vi "TCPserver.vi"(11 "Ref In":T1) -> ()   [LabVIEW 2016]
doc: "Demonstrates how to open a connection to an TCP server, read the data being sent, and display the data on a chart. This VI is designed to stop if the TCP connection is terminated."
panel:
  out "error out":errorcluster
  out "Current Pos":dbl[](array[numeric])
  in  "Position":dbl[](array[numeric])
  in  "Ring":u16(ring) items=["Move2Pos", "Move2Work", "ChangeManipulator", "Move2Home", "Calibration", "CurrentPos", "Interrupt"]
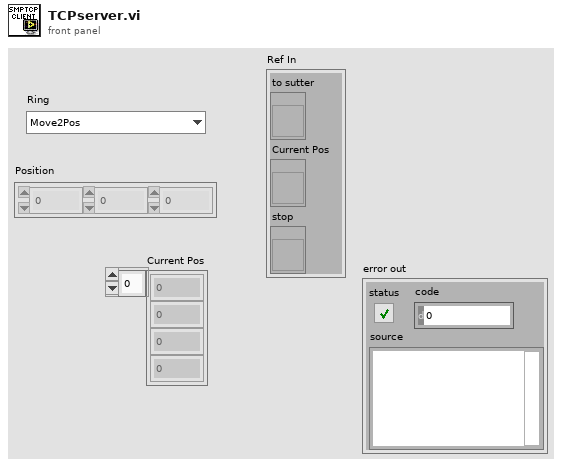
[diagram p1: front panel]
types:
  T1 = cluster{"to sutter":refnum<vi>, "Current Pos":refnum<vi>, "stop":refnum<vi>}
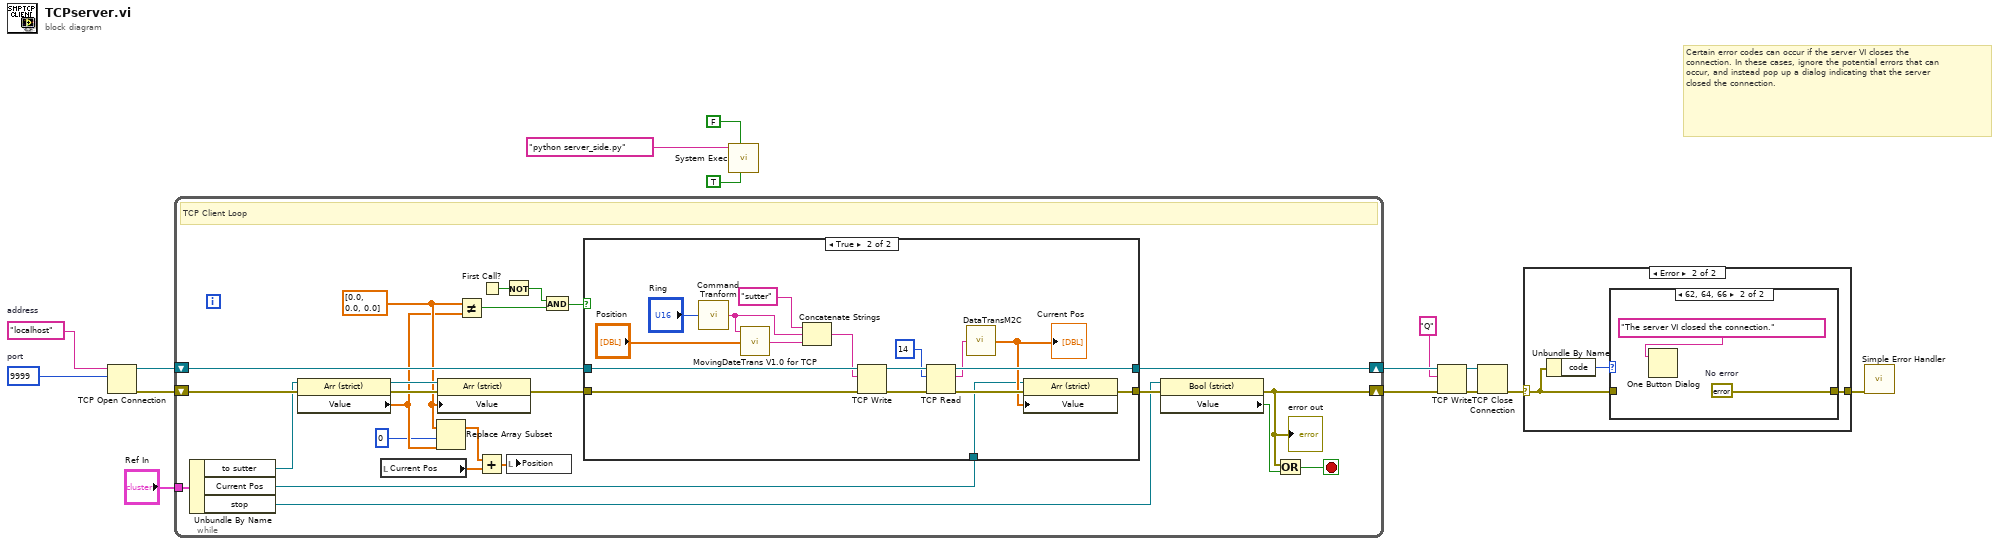
[diagram p0: block diagram]
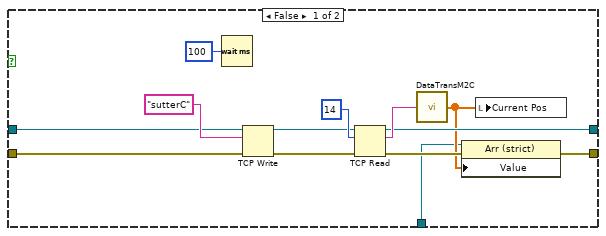
[diagram p4: hidden frame]
diagram:
  w7 = u16 9999  # port
  w8 = "localhost"  # address
  # "Certain error codes can occur if the server VI closes the connection. In these cases, ignore the potential errors that can occur, and instead pop up a dialog indicating that the server closed the connection."
  n1 = TCP Open Connection(address=w8, remote port or service name=w7) -> (connection ID=w5:refnum<k5>, error out=w4:errorcluster)  [unwired: 3 in]
  n2 = while {
    shift-right: [w34] -> w12
    shift-left: w4 -> [w39]
    shift-right: [w36] -> w14
    shift-left: w5 -> [w37]
    tunnel: "Ref In" -> [w27]
    stop <- w38 stop-if-true
    w19 = dbl[] [0.0, 0.0, 0.0] ("x")
    # "TCP Client Loop"
    n3 = Unbundle By Name(w27) -> ("to sutter"=w32:refnum<vi>, "Current Pos"=w20:refnum<vi>, "stop"=w21:refnum<vi>)
    n4 = property class="Arr (strict)"(reference=w32, error in=w39) -> (reference out=w30:refnum<vi>, error out=w29:errorcluster, "Value"=w18:sgl[])
    n5 = local read "Current Pos"() -> (w31:dbl[])
    n6 = Replace Array Subset(array=w19, new element=w18, index=0) -> (w17:dbl[])
    n7 = property class="Arr (strict)"(reference=w30, error in=w29, "Value"=w19) -> (error out=w28:errorcluster)  [unwired: 1 out]
    n8 = Not Equal?(x=w19, y=w18) -> (x != y?=w23:bool)
    n9 = Add(x=w17, y=w31) -> (x+y=w26:dbl[])
    n10 = First Call?() -> (First Call?: T/F=w25:bool)
    n11 = Not(x=w25) -> (.not. x?=w24:bool)
    n12 = local write "Position"(w26) -> ()
    n13 = And(x=w24, y=w23) -> (x .and. y?=w22:bool)
    n14 = case shown="True" w22 {
      tunnel: w37 -> [w46 w69]
      tunnel: [w44 w68] -> w36
      tunnel: [w42 w55] -> w35
      tunnel: w28 -> [w45 w57]
      tunnel: w20 -> [w40 w53]
      frame False {
        n15 = Wait (ms)(milliseconds to wait=u32 100) -> ()  [unwired: 1 out]
        n16 = TCP Write(connection ID=w46, data in="sutterC", error in (no error)=w45) -> (connection ID out=w49:refnum<k5>, error out=w48:errorcluster)  [unwired: 1 in, 1 out]
        n17 = TCP Read(connection ID=w49, bytes to read=14, error in (no error)=w48) -> (connection ID out=w44:refnum<k5>, data out=w51:string, error out=w43:errorcluster)  [unwired: 2 in]
        n18 = call "DataTransM2C.vi"("MotorData"=w51) -> ("Computer Data"=w41:dbl[])
        n19 = property class="Arr (strict)"(reference=w40, error in=w43, "Value"=w41) -> (error out=w42:errorcluster)  [unwired: 1 out]
        n20 = local write "Current Pos"(w41) -> ()
      }
      frame True {
        n21 = call "Command Tranform.vi"("Command"="Ring") -> ("command str"=w64:string)
        n22 = call "MovingDateTrans V1.0 for TCP.vi"("INPUT"="Position", "String"=w64) -> ("MOVEING COMMAND"=w66:string)  [unwired: 1 in]
        n23 = Concatenate Strings("sutter" ("string"), w64, w66) -> (w59:string)
        n24 = TCP Write(connection ID=w69, data in=w59, error in (no error)=w57) -> (connection ID out=w62:refnum<k5>, error out=w63:errorcluster)  [unwired: 1 in, 1 out]
        n25 = TCP Read(connection ID=w62, bytes to read=14, error in (no error)=w63) -> (connection ID out=w68:refnum<k5>, data out=w60:string, error out=w56:errorcluster)  [unwired: 2 in]
        n26 = call "DataTransM2C.vi"("MotorData"=w60) -> ("Computer Data"=w54:dbl[])
        "Current Pos" <- w54
        n27 = property class="Arr (strict)"(reference=w53, error in=w56, "Value"=w54) -> (error out=w55:errorcluster)  [unwired: 1 out]
      }
    }
    n28 = property class="Bool (strict)"(reference=w21, error in=w35) -> (error out=w34:errorcluster, "Value"=w33:bool)  [unwired: 1 out]
    "error out" <- w34
    n29 = Or(x=w34, y=w33) -> (x .or. y?=w38:bool)
  }
  n30 = call <vilib>:"System Exec.vi"("run minimized? (F)"=TRUE, "wait until completion? (T)"=FALSE, "command line"="python server_side.py") -> ()  [unwired: 5 in, 4 out]
  n31 = TCP Write(connection ID=w14, data in="Q", error in (no error)=w12) -> (connection ID out=w15:refnum<k5>, error out=w13:errorcluster)  [unwired: 2 out]
  n32 = TCP Close Connection(connection ID=w15, error in (no error)=w13) -> (error out=w10:errorcluster)  [unwired: 1 in, 1 out]
  n33 = case shown="Error" w10 {
    selector: w10 -> [w70 w72]
    tunnel: [w70 w71] -> w9
    frame No Error {
    }
    frame Error {
      n34 = Unbundle By Name(w72) -> ("code"=w73:i32)
      n35 = case shown="62, 64, 66" w73 {
        tunnel: w72 -> [w74 _]
        tunnel: [w74 w76] -> w71
        frame Default {
        }
        frame 62, 64, 66 {
          w76 = errorcluster {"status"=FALSE, "code"=0, "source"=""}  # No error
          n36 = One Button Dialog(message="The server VI closed the connection.") -> ()  [unwired: 1 in, 1 out]
        }
      }
    }
  }
  n37 = call <vilib>:"Simple Error Handler.vi"("error in (no error)"=w9) -> ()  [unwired: 4 in, 5 out]
